vi "LoadSettings2.vi"(8 "error in (no error)":errorcluster, 11 "Settings In":T1={"Harware Configuration"={"Camera"="cam2", "Frames Per Second"=15, "Simulate Recording"=TRUE, "Simulated Recording Sample"=path "D:/Dropbox/MyPrograms/LabViewLibraries/ImageAcquisitionProgram/SimulationInput/SampleImage.jpg", "Timestamp Method"=enum."Camera Timestamp"}, "Base Recording Path"=path "", "Type Of Recording"="", "Recording Codec"="", "TrackingSettings"={"Max Radius"=10, "Threshold"=0.0, "ROI"={"Left"=1, "Top"=1, "Right"=424, "Bottom"=512, "Rotation"=0.0}}, "Calibration"={"Pixel Width (X)"=1.0, "Pixel Height (Y)"=1.0}, "Broadcast Length"=1} {"Broadcast Length" min=0; "TrackingSettings"."ROI"."Rotation" format="%.2f"; "TrackingSettings"."ROI"."Left" scale=0.0..1024.0; "TrackingSettings"."ROI"."Right" scale=0.0..1024.0; "TrackingSettings"."Threshold" scale=0.0..255.0}) -> (0 "error out":errorcluster, 3 "Settings Out":T1={"Harware Configuration"={"Camera"="cam1", "Frames Per Second"=15, "Simulate Recording"=FALSE, "Simulated Recording Sample"=path "", "Timestamp Method"=enum."Camera Timestamp"}, "Base Recording Path"=path "", "Type Of Recording"="", "Recording Codec"="", "TrackingSettings"={"Max Radius"=0, "Threshold"=160.0, "ROI"={"Left"=0, "Top"=0, "Right"=0, "Bottom"=0, "Rotation"=0.0}}, "Calibration"={"Pixel Width (X)"=1.0, "Pixel Height (Y)"=1.0}, "Broadcast Length"=0} {"Broadcast Length" min=0; "TrackingSettings"."ROI"."Rotation" format="%.2f"; "TrackingSettings"."ROI"."Left" scale=0.0..1024.0; "TrackingSettings"."ROI"."Right" scale=0.0..1024.0; "TrackingSettings"."Threshold" scale=0.0..255.0})   [LabVIEW 2017, in "ImageAcquisitionLibrary.lvlib"]
uses:
  ImageAcquisitionLibrary.lvlib
  Settings.ctl
  <vilib>/userdefined/High Color/IMAQdx.ctl
  Tracking/TrackingSettings.ctl
  Calibration.ctl
  <vilib>/Utility/xml.llb/Read From XML File(string).vi
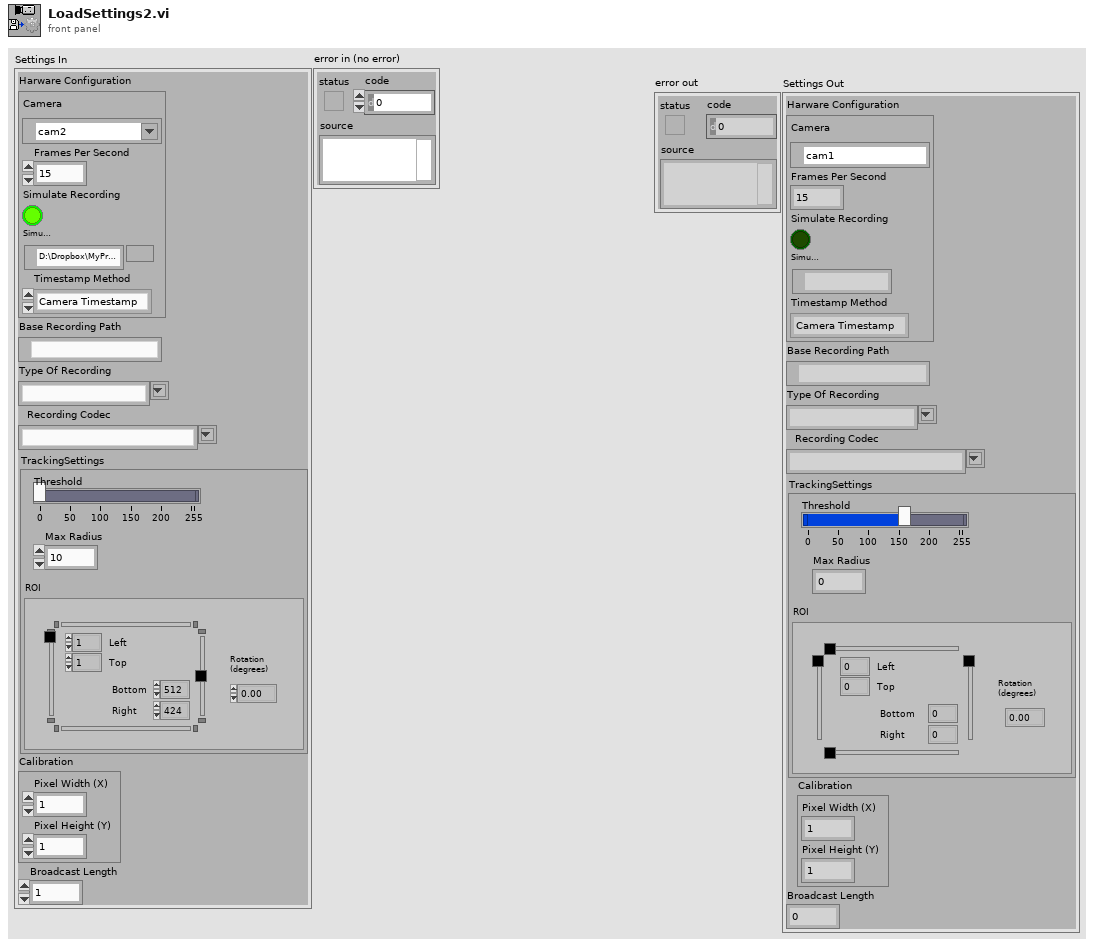
[diagram p1: front panel]
types:
  T1 = typedef "ImageAcquisitionLibrary.lvlib/Settings.ctl" = cluster{"Harware Configuration":cluster{"Camera":T2, "Frames Per Second":u32, "Simulate Recording":bool, "Simulated Recording Sample":path, "Timestamp Method":enum16{"System Timestamp", "Camera Timestamp", "IMAQdx Timestamp"}}, "Base Recording Path":path, "Type Of Recording":string, "Recording Codec":string, "TrackingSettings":T3, "Calibration":T5, "Broadcast Length":i32}
  T2 = typedef "IMAQdx.ctl" = refnum<k21>
  T3 = typedef "ImageAcquisitionLibrary.lvlib/TrackingSettings.ctl" = cluster{"Max Radius":i32, "Threshold":sgl, "ROI":T4}
  T4 = typedef "IMAQ Rectangle" = cluster{"Left":i32, "Top":i32, "Right":i32, "Bottom":i32, "Rotation":dbl}
  T5 = typedef "ImageAcquisitionLibrary.lvlib/Calibration.ctl" = cluster{"Pixel Width (X)":dbl, "Pixel Height (Y)":dbl}
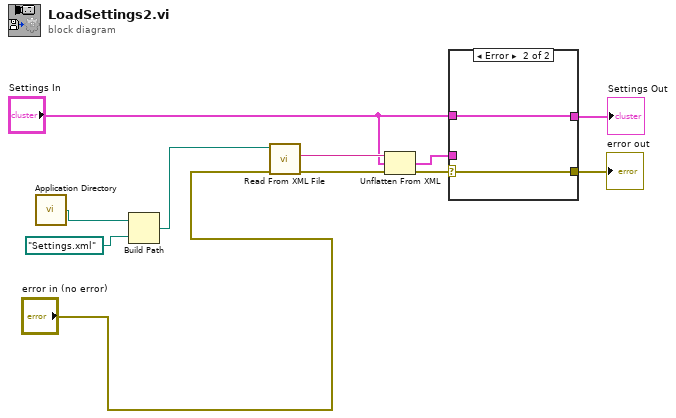
[diagram p0: block diagram]
diagram:
  n1 = call <vilib>:"Application Directory.vi"() -> ("Application Directory"=w10:path)
  n2 = Build Path(base path=w10, name or relative path=path "Settings.xml" ("base path")) -> (appended path=w9:path)
  n3 = call-poly <vilib>:"Read From XML File.vi"("error in (no error)"="error in (no error)", "XML File Path"=w9) -> ("error out"=w5:errorcluster, "XML Elements"=w3:string)  [unwired: 7 in, 1 out]
  n4 = Unflatten From XML(xml string=w3, type="Settings In", error in (no error)=w5) -> (value=w1:T1, error out=w4:errorcluster)
  n5 = case shown="Error" w4 {
    selector: w4 -> [w13 w14]
    tunnel: "Settings In" -> [_ w15]
    tunnel: [w12 w15] -> w8
    tunnel: [w13 w14] -> w7
    tunnel: w1 -> [w12 _]
    frame No Error {
    }
    frame Error {
    }
  }
  "Settings Out" <- w8
  "error out" <- w7
